vi "Close Example Device.vi"(11 "ExampleDevice.lvclass":refnum<class "ExampleDevice.lvclass">) -> (3 "ExampleDevice.lvclass 2":refnum<class "ExampleDevice.lvclass">)   [LabVIEW 2023, in "ExampleDevice.lvclass"]
uses:
  ExampleDevice.lvclass
  ExampleDevice.lvclass/ExampleDevice.ctl
  Setpoint/Setpoint.lvclass
  Current Setpoint/Current Setpoint.lvclass
  D:/Labview/bls-capabilities-bto/Setpoint/Setpoint.lvclass
  D:/Labview/bls-capabilities-bto/Current Setpoint/Current Setpoint.lvclass
  Voltage Setpoint/Voltage Setpoint.lvclass
  D:/Labview/bls-capabilities-bto/Voltage Setpoint/Voltage Setpoint.lvclass
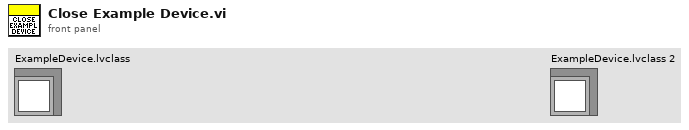
[diagram p1: front panel]
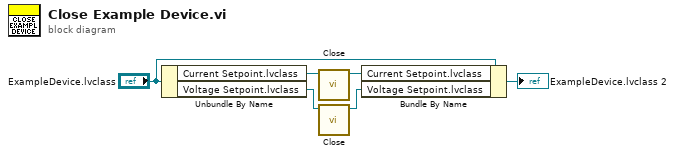
[diagram p0: block diagram]
diagram:
  n1 = Unbundle By Name("ExampleDevice.lvclass") -> ("Current Setpoint.lvclass"=w4:refnum<class "Current Setpoint.lvclass">, "Voltage Setpoint.lvclass"=w2:refnum<class "Voltage Setpoint.lvclass">)
  n2 = call "Close.vi"("Setpoint.lvclass"=w4) -> ("Setpoint.lvclass 2"=w3:refnum<class "Current Setpoint.lvclass">)  [unwired: 9 in, 1 out]
  n3 = call "Close.vi"("Setpoint.lvclass"=w2) -> ("Setpoint.lvclass 2"=w1:refnum<class "Voltage Setpoint.lvclass">)  [unwired: 9 in, 1 out]
  n4 = Bundle By Name(cluster="ExampleDevice.lvclass", "Current Setpoint.lvclass"=w3, "Voltage Setpoint.lvclass"=w1) -> (→"ExampleDevice.lvclass 2":refnum<class "ExampleDevice.lvclass">)
